vi "Remove Ports.vi"(8 "error in":errorcluster, 9 "refresh?":bool=TRUE, 11 "Custom device Ref":T1 format="%.0x") -> (0 "error out":errorcluster, 3 "Custom device Ref out":T1 format="%.0x")   [LabVIEW 2020, in "AIM ARINC 664 Scripting.lvlib"]
uses:
  AIM ARINC 664 Scripting.lvlib
  <vilib>/NI VeriStand/Custom Device API/Custom Device Item Ref.ctl
  <vilib>/NI/VeriStand Custom Device Serialization/System Explorer Action.ctl
  Constants.vi
  <vilib>/NI VeriStand/Custom Device Tools/Custom Device Utility Library/NI VeriStand - Search for Item by GUID.vi
  <vilib>/NI VeriStand/Custom Device Tools/Custom Device Utility Library/Custom Device Utility Library.lvlib
  <vilib>/NI VeriStand/Custom Device API/Custom Device API.lvlib
  <vilib>/NI/VeriStand Custom Device Serialization/Custom Device Serialization.lvlib
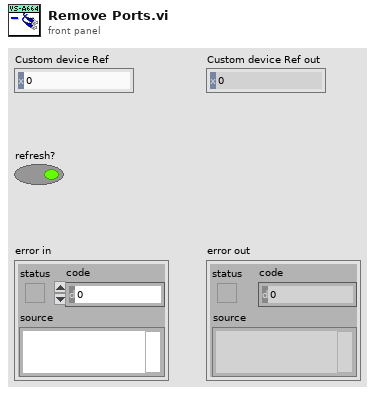
[diagram p1: front panel]
types:
  T1 = typedef "Custom Device API.lvlib/Custom Device Item Ref.ctl" = u64
  T2 = typedef "Custom Device Serialization.lvlib/System Explorer Action.ctl" = u16
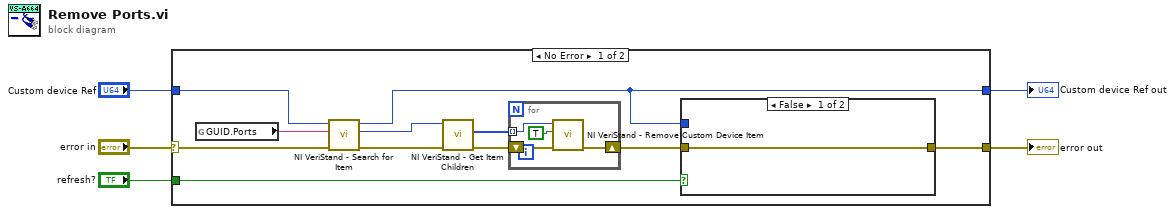
[diagram p0: block diagram]
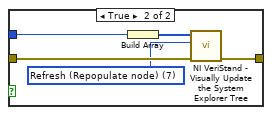
[diagram p2: hidden frame]
diagram:
  n1 = case shown="No Error" "error in" {
    selector: "error in" -> [w15 w28]
    tunnel: "Custom device Ref" -> [w16 w27]
    tunnel: [w8 w28] -> w4
    tunnel: [w7 w27] -> w3
    tunnel: "refresh?" -> [w6 _]
    frame No Error {
      n2 = global read "Constants.vi" "GUID.Ports"() -> (w14:string)
      n3 = call-poly <vilib>:"NI VeriStand - Search for Item.vi"("error in"=w15, "Item GUID"=w14, "Section Ref in"=w16) -> ("error out"=w11:errorcluster, "Item Ref"=w12:T1, "Section Ref out"=w7:T1)  [unwired: 5 in, 1 out]
      n4 = call <vilib>:"NI VeriStand - Get Item Children.vi"("error in (no error)"=w11, "Item Ref in"=w12) -> ("error out"=w10:errorcluster, "Child Refs"=w9:T1[])  [unwired: 6 in, 2 out]
      n5 = for {
        shift-right: [w26] -> w13
        shift-left: w10 -> [w24]
        tunnel: w9 -> [w23] mode=indexing
        n6 = call <vilib>:"NI VeriStand - Remove Custom Device Item.vi"("error in (no error)"=w24, "Force Delete (F)"=TRUE, "Item Ref in"=w23) -> ("error out"=w26:errorcluster)  [unwired: 7 in, 1 out]
      }
      n7 = case shown="False" w6 {
        tunnel: w13 -> [w17 w22]
        tunnel: [w17 w21] -> w8
        tunnel: w7 -> [_ w20]
        frame False {
        }
        frame True {
          w18 = T2 7 items=["Refresh (Add)"=5, "Refresh (Repopulate node)"=7] ("Action")
          n8 = Build Array(w20) -> (w19:T1[])
          n9 = call <vilib>:"NI VeriStand - Visually Update the System Explorer Tree.vi"("error in (no error)"=w22, "Action"=w18, "Node IDs"=w19) -> ("error out"=w21:errorcluster)  [unwired: 8 in]
        }
      }
    }
    frame Error {
    }
  }
  "error out" <- w4
  "Custom device Ref out" <- w3
